vi "E4440A_PSA_Defaults.vi"(8 "error in (no error)":errorcluster, 11 "VISA resource name":refnum<visa-resource-name>) -> (0 "error out":errorcluster, 3 "VISA resource name out":refnum<visa-resource-name>)   [LabVIEW 2015]
doc: "This Utility VI sends a default command string to the instrument whenever a new VISA session is opened, or the instrument is reset. Use this VI as a subVI for the Initialize and Reset VIs. Altering this VI could cause these two VIs to operate incorrectly."
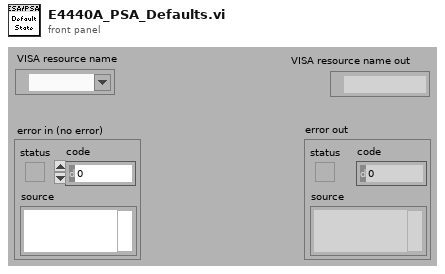
[diagram p1: front panel]
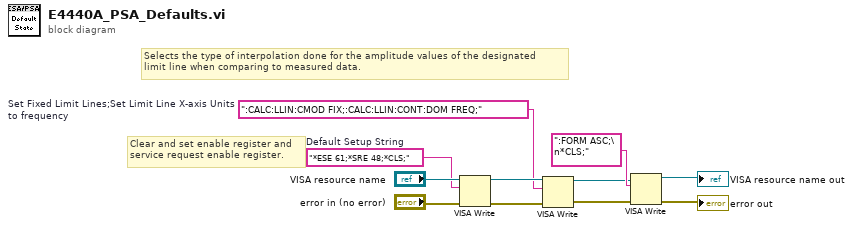
[diagram p0: block diagram]
diagram:
  w6 = ":CALC:LLIN:CMOD FIX;:CALC:LLIN:CONT:DOM FREQ;"  # Set Fixed Limit Lines;Set Limit Line X-axis Units to frequency
  w9 = "*ESE 61;*SRE 48;*CLS;"  # Default Setup String
  # "Selects the type of interpolation done for the amplitude values of the designated\nlimit line when comparing to measured data."
  # "Clear and set enable register and \nservice request enable register."
  n1 = VISA Write(VISA resource name="VISA resource name", write buffer=w9, error in (no error)="error in (no error)") -> (VISA resource name out=w7:refnum<visa-resource-name>, error out=w8:errorcluster)  [unwired: 1 out]
  n2 = VISA Write(VISA resource name=w7, write buffer=w6, error in (no error)=w8) -> (VISA resource name out=w4:refnum<visa-resource-name>, error out=w3:errorcluster)  [unwired: 1 out]
  n3 = VISA Write(VISA resource name=w4, write buffer=":FORM ASC;\n*CLS;" ("Fetch Measurement"), error in (no error)=w3) -> (VISA resource name out=→"VISA resource name out":refnum<visa-resource-name>, error out=→"error out":errorcluster)  [unwired: 1 out]
